vi "Button press.vi"(11 "Boolean":bool) -> (3 "Boolean 2":bool)   [LabVIEW 2016]
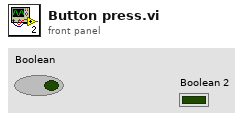
[diagram p1: front panel]
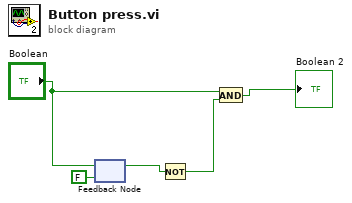
[diagram p0: block diagram]
diagram:
  n1 = feedback-in #1("Boolean") -> ()
  n2 = feedback #1(FALSE ("Boolean")) -> (w4:bool)
  n3 = Not(x=w4) -> (.not. x?=w3:bool)
  n4 = And(x="Boolean", y=w3) -> (x .and. y?=→"Boolean 2":bool)
